vi "Async.vi"(6 "Reconnect Parameters":T1={"IP Address"="", "JSON"="", "bytes to read (1024)"=1024, "timeout ms (5)"=5, "port (4222)"=4222}, 7 "error queue":refnum<queue>, 8 "sub map":refnum<data-value>, 9 "subscriptions queue":refnum<queue>, 10 "async stop notifier":refnum<notifier>, 11 "NATS Connection":refnum<data-value>) -> ()   [LabVIEW 2024, in "NATS Client.lvlib" / "NATS Client.lvclass"]
doc: "Reads a message from the NATS server."
uses:
  NATS Client.lvclass
  subscription queue.ctl
  subscription actions.ctl
  NATS Subscription/NATS Subscription.lvclass
  <vilib>/NATS/NATS Core/Controls/nats connection.ctl
  Reconnect Parameters.ctl
  Subscription Map.ctl
  NATS Client.lvclass/NATS Client.ctl
  <vilib>/NATS/NATS Core/NATS Core.lvlib
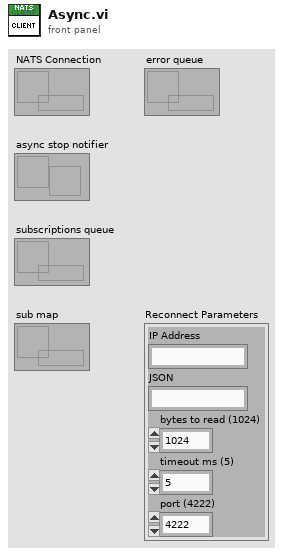
[diagram p1: front panel]
types:
  T1 = typedef "NATS Client.lvlib/NATS Client.lvclass/Reconnect Parameters.ctl" = cluster{"IP Address":string, "JSON":string, "bytes to read (1024)":i32, "timeout ms (5)":i32, "port (4222)":u16}
  T2 = typedef "NATS Client.lvlib/NATS Client.lvclass/Subscription Map.ctl" = map{string, refnum<class "NATS Subscription.lvclass">}
  T3 = typedef "NATS Core.lvlib/nats connection.ctl" = cluster{"connection ID":refnum<k5>, "server INFO":string, "timeout ms":i32, "verbose?":bool, "server headers?":bool, "client headers?":bool}
  T4 = typedef "NATS Core.lvlib/nats message.ctl" = cluster{"subject":string, "payload":string, "sub id":string, "reply-to":string, "headers":string, "type":T5, "received":timestamp}
  T5 = typedef "NATS Core.lvlib/msg type.ctl" = enum16{"Undefined", "MSG", "HMSG", "+OK", "PING", "PONG", "-ERR", "INFO"}
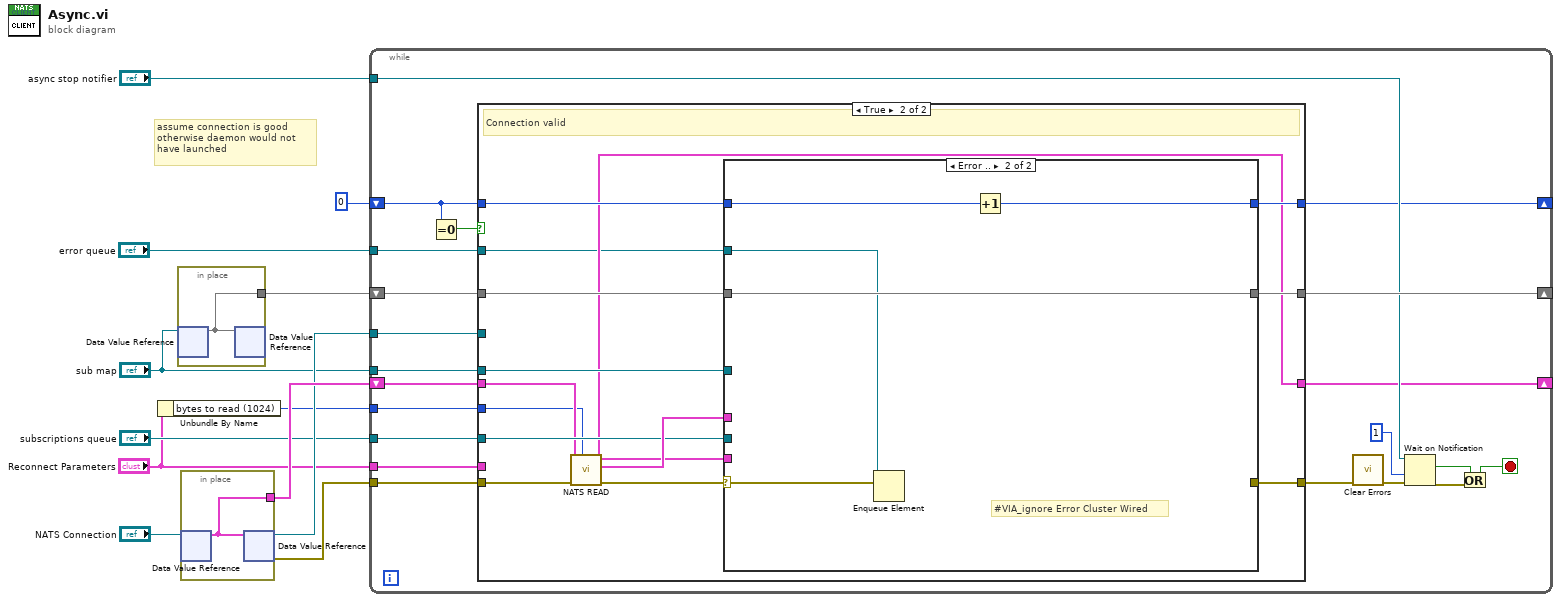
[diagram p0: block diagram]
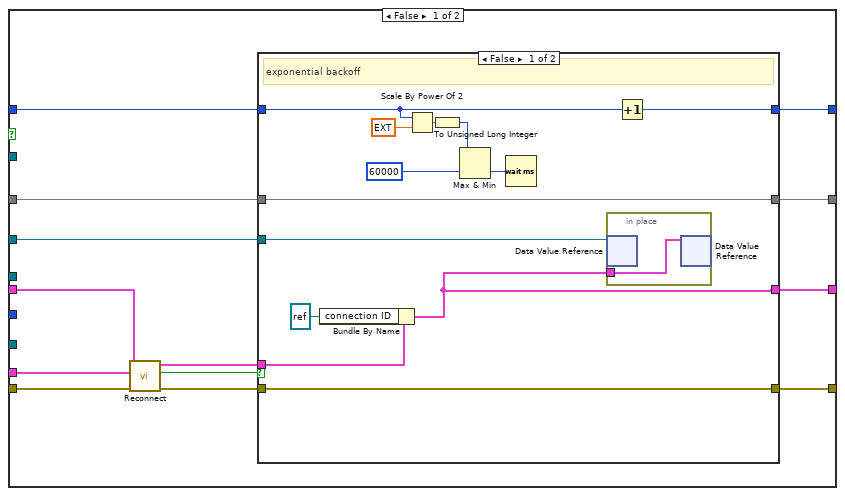
[diagram p2: hidden frame]
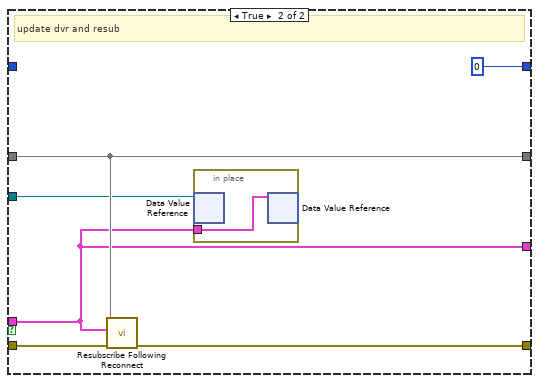
[diagram p3: hidden frame]
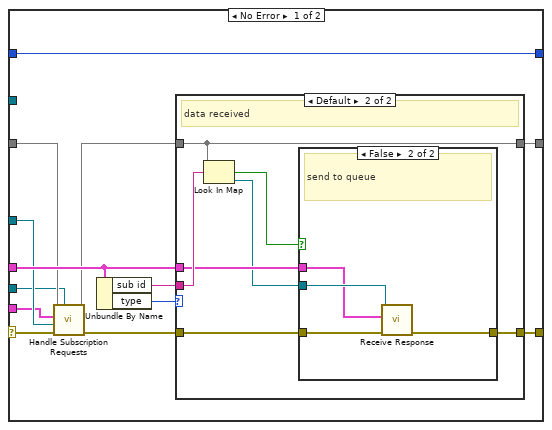
[diagram p4: hidden frame]
diagram:
  # "assume connection is good\notherwise daemon would not \nhave launched"
  n1 = Unbundle By Name("Reconnect Parameters") -> ("bytes to read (1024)"=w1:i32)
  n2 = in-place {
    in-place-border: [w13] -> w6
    n3 = in-place-dvr #1("sub map") -> (w13:T2)  [unwired: 1 out]
    n4 = in-place-dvr #1(w13) -> ()  [unwired: 2 out]
  }
  n5 = in-place {
    in-place-border: [w14] -> w10
    n6 = in-place-dvr #2("NATS Connection") -> (w14:T3)  [unwired: 1 out]
    n7 = in-place-dvr #2(w14) -> (w8:refnum<data-value>, w11:errorcluster)
  }
  n8 = while {
    shift-right: [w34] -> _
    shift-left: w6 -> [w29]
    tunnel: "async stop notifier" -> [w32]
    tunnel: w8 -> [w20]
    shift-right: [w19] -> _
    shift-left: w10 -> [w23]
    shift-right: [w31] -> _
    shift-left: u32 0 -> [w25]
    tunnel: "sub map" -> [w28]
    tunnel: "error queue" -> [w18]
    tunnel: "subscriptions queue" -> [w27]
    tunnel: "Reconnect Parameters" -> [w22]
    tunnel: w1 -> [w21]
    tunnel: w11 -> [w24]
    stop <- w15 stop-if-true
    n9 = Equal To 0?(x=w25) -> (x = 0?=w26:bool)
    n10 = case shown="True" w26 {
      tunnel: [w39 w83] -> w34
      tunnel: [w44 w80] -> w31
      tunnel: w25 -> [w38 w79]
      tunnel: [w40 w78] -> w30
      tunnel: w29 -> [w42 w77]
      tunnel: w28 -> [_ w76]
      tunnel: w27 -> [_ w75]
      tunnel: w24 -> [w48 w74]
      tunnel: w23 -> [w47 w73]
      tunnel: w22 -> [w46 _]
      tunnel: w21 -> [_ w72]
      tunnel: w20 -> [w37 _]
      tunnel: [w36 w71] -> w19
      tunnel: w18 -> [_ w70]
      frame False {
        n11 = call "Reconnect.vi"("error in"=w48, "Reconnect Parameters"=w46, "nats connection in"=w47) -> ("error out"=w43:errorcluster, "CONNECT processed?"=w45:bool, "nats connection out"=w41:T3)  [unwired: 6 in]
        n12 = case shown="False" w45 {
          tunnel: [w60 u32 0] -> w44
          tunnel: w43 -> [w53 w67]
          tunnel: w42 -> [w61 w65]
          tunnel: w41 -> [w51 w63]
          tunnel: [w53 w66] -> w40
          tunnel: [w61 w65] -> w39
          tunnel: w38 -> [w55 _]
          tunnel: w37 -> [w52 w64]
          tunnel: [w50 w63] -> w36
          frame False {
            # "exponential backoff"
            n13 = Bundle By Name(cluster=w51, "connection ID"=refnum<k5> refnum) -> (w50:T3)
            n14 = Scale By Power Of 2(n=w55, x=ext 100.0) -> (x*2^n=w58:ext)
            n15 = To Unsigned Long Integer(number=w58) -> (unsigned 32bit integer=w59:u32)
            n16 = Max & Min(x=w59, y=u32 60000) -> (min(x,y)=w57:u32)  [unwired: 1 out]
            n17 = Wait (ms)(milliseconds to wait=w57) -> ()  [unwired: 1 out]
            n18 = in-place {
              in-place-border: w50 -> [w62]
              n19 = in-place-dvr #3(w52) -> ()  [unwired: 2 out]
              n20 = in-place-dvr #3(w62) -> ()  [unwired: 2 out]
            }
            n21 = Increment(x=w55) -> (x+1=w60:u32)
          }
          frame True {
            # "update dvr and resub"
            n22 = call "Resubscribe Following Reconnect.vi"("error in"=w67, "nats connection in"=w63, "subs in"=w65) -> ("error out"=w66:errorcluster)  [unwired: 8 in]
            n23 = in-place {
              in-place-border: w63 -> [w69]
              n24 = in-place-dvr #4(w64) -> ()  [unwired: 2 out]
              n25 = in-place-dvr #4(w69) -> ()  [unwired: 2 out]
            }
          }
        }
      }
      frame True {
        # "Connection valid"
        n26 = call <vilib>:"NATS READ.vi"("bytes to read (1024)"=w72, "error in"=w74, "nats connection in"=w73) -> ("error out"=w81:errorcluster, "nats message"=w82:T4, "nats connection out"=w71:T3)  [unwired: 5 in, 1 out]
        n27 = case shown="Error .." w81 {
          selector: w81 -> [w90 w113]
          tunnel: [w96 _] -> w78
          tunnel: [w94 w115] -> w83
          tunnel: w77 -> [w87 w115]
          tunnel: w82 -> [w92 _]
          tunnel: w71 -> [w84 _]
          tunnel: [w91 w111] -> w80
          tunnel: w79 -> [w91 w114]
          tunnel: w76 -> [w86 _]
          tunnel: w75 -> [w85 _]
          tunnel: w70 -> [_ w112]
          frame No Error {
            n28 = call "Handle Subscription Requests.vi"("subscriptions queue"=w85, "error in"=w90, "sub map"=w86, "nats connection in"=w84, "subs in"=w87) -> ("error out"=w89:errorcluster, "subs out"=w88:T2)  [unwired: 5 in]
            n29 = Unbundle By Name(w92) -> ("sub id"=w95:string, "type"=w93:T5)
            n30 = case shown="Default" w93 {
              tunnel: w89 -> [w98 w105]
              tunnel: w95 -> [_ w103]
              tunnel: w88 -> [w97 w102]
              tunnel: [w97 w102] -> w94
              tunnel: [w98 w104] -> w96
              tunnel: w92 -> [_ w100]
              frame "Undefined" {
              }
              frame Default {
                # "data received"
                n31 = Look In Map(map=w102, key=w103) -> (key not found?=w101:bool, value=w99:refnum<class "NATS Subscription.lvclass">)  [unwired: 1 in]
                n32 = case shown="False" w101 {
                  tunnel: w105 -> [w106 w110]
                  tunnel: [w106 w109] -> w104
                  tunnel: w100 -> [_ w107]
                  tunnel: w99 -> [_ w108]
                  frame True {
                  }
                  frame False {
                    # "send to queue"
                    n33 = call "Receive Response.vi"("error in"=w110, "nats message"=w107, "NATS Subscriber in"=w108) -> ("error out"=w109:errorcluster)  [unwired: 7 in, 1 out]
                  }
                }
              }
            }
          }
          frame Error {
            # "#VIA_ignore Error Cluster Wired"
            n34 = Enqueue Element(queue=w112, element=w113) -> ()  [unwired: 2 in, 3 out]
            n35 = Increment(x=w114) -> (x+1=w111:u32)
          }
        }
      }
    }
    n36 = call <vilib>:"Clear Errors.vi"("error in (no error)"=w30) -> ("error out"=w35:errorcluster)  [unwired: 5 in, 1 out]
    n37 = Wait on Notification(notifier=w32, timeout in ms (-1)=1, error in (no error)=w35) -> (notification=w16:bool, error out=w17:errorcluster)  [unwired: 1 in, 2 out]
    n38 = Or(x=w16, y=w17) -> (x .or. y?=w15:bool)
  }
